vi "Module Type.vi"(11 "GenericGuiAI in":refnum<class "GenericGuiAI.lvclass">) -> (2 "Module Type":string)   [LabVIEW 2020, in "VolatusDAQGenericGUI.lvlib" / "GenericGuiAI.lvclass"]
uses:
  GenericGuiAI.lvclass
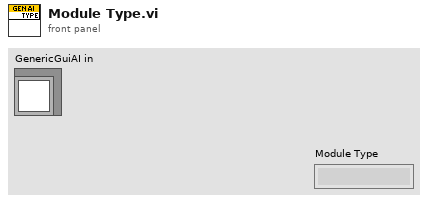
[diagram p1: front panel]
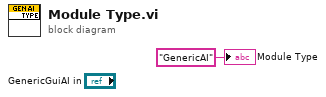
[diagram p0: block diagram]
diagram:
  "Module Type" <- "GenericAI" ("Module Type")
